vi "n prime numbers.vi"() -> ()   [LabVIEW 2020]
panel:
  out "Array":string[][](array[string])
  in  "Numeric":dbl
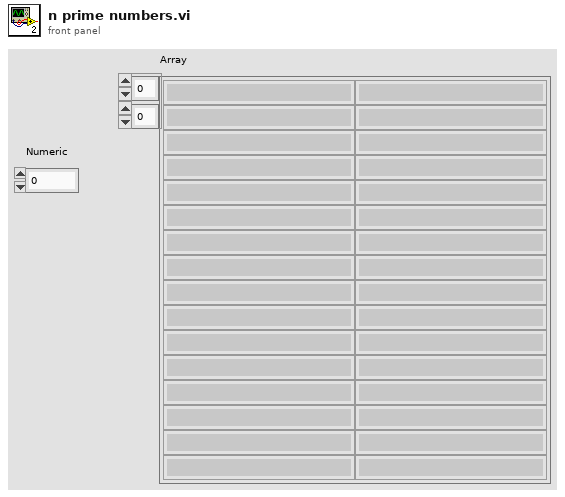
[diagram p1: front panel]
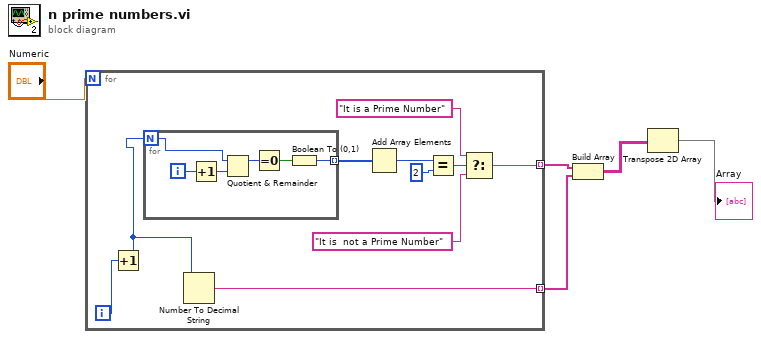
[diagram p0: block diagram]
diagram:
  n1 = for {
    N: "Numeric" -> [_]
    tunnel: [w8] -> w5 mode=indexing
    tunnel: [w7] -> w3 mode=indexing
    i -> [w9]
    n2 = Increment(x=w9) -> (x+1=w6:i32)
    n3 = for {
      N: w6 -> [w19]
      tunnel: [w17] -> w15 mode=indexing
      i -> [w21]
      n4 = Increment(x=w21) -> (x+1=w20:i32)
      n5 = Quotient & Remainder(x=w19, y=w20) -> (x-y*floor(x/y)=w16:i32)  [unwired: 1 out]
      n6 = Equal To 0?(x=w16) -> (x = 0?=w18:bool)
      n7 = Boolean To (0,1)(Boolean=w18) -> (0, 1=w17:i16)
    }
    n8 = Number To Decimal String(number=w6) -> (decimal integer string=w7:string)  [unwired: 1 in]
    n9 = Add Array Elements(numeric array=w15) -> (sum=w14:i16)
    n10 = Equal?(x=w14, y=i16 2) -> (x = y?=w12:bool)
    n11 = Select(t="It is a Prime Number", s=w12, f="It is  not a Prime Number") -> (s? t:f=w8:string)
  }
  n12 = Build Array(w5, w3) -> (w2:string[][])
  n13 = Transpose 2D Array(2D array=w2) -> (transposed array=→"Array":string[][])
